vi "GetType.vi"(8 "error in (no error)":errorcluster, 11 "Reset Device Msg":refnum<class "Reset Device Msg.lvclass">) -> (0 "error out":errorcluster, 2 "Data Sample":variant, 3 "Reset Device Msg":refnum<class "Reset Device Msg.lvclass">)   [LabVIEW 2015, in "CS++DeviceActor.lvlib" / "Reset Device Msg.lvclass"]
doc: "This VI delivers a sample of the data type format the message expects."
uses:
  Reset Device Msg.lvclass
  Reset Device Msg.lvclass/Reset Device Msg.ctl
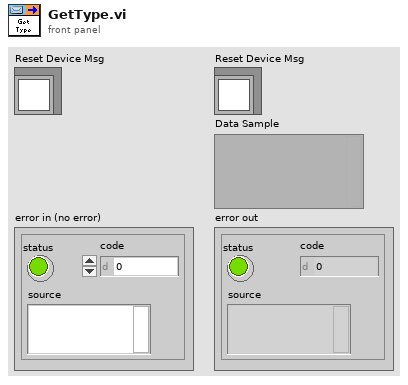
[diagram p1: front panel]
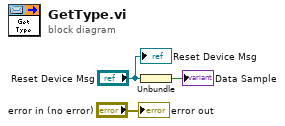
[diagram p0: block diagram]
diagram:
  n1 = Unbundle("Reset Device Msg") -> (→"Data Sample":bool)
  "error out" <- "error in (no error)"
  "Reset Device Msg" <- "Reset Device Msg"
